vi "Overlay Arrow on Arc.vi"(5 "End Angle (degrees)":dbl format="%.2f", 6 "Scan Direction":u32(ring) items=["Counter-Clockwise", "Clockwise"], 7 "Start Angle (degrees)":dbl format="%.2f", 8 "error in (no error)":errorcluster, 9 "Color":u32(colorbox)=16711680, 10 "Bounding Rectangle":T2, 11 "Image":T1) -> (0 "error out":errorcluster, 3 "Image Out":T1)   [LabVIEW 2020]
uses:
  IMAQ Image.ctl
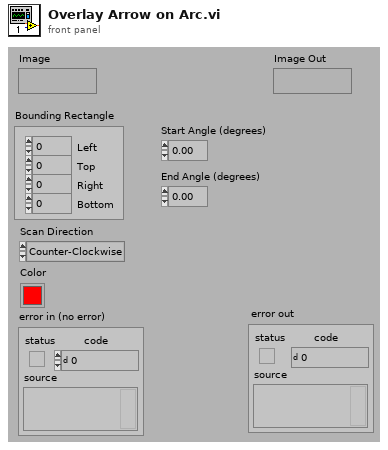
[diagram p1: front panel]
types:
  T1 = typedef "IMAQ Image.ctl" = refnum<image>
  T2 = cluster{"Left":i32, "Top":i32, "Right":i32, "Bottom":i32}
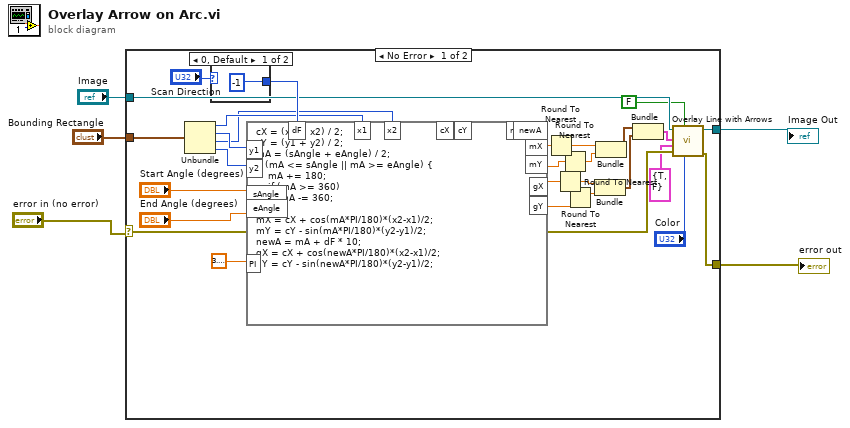
[diagram p0: block diagram]
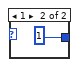
[diagram p2: hidden frame]
diagram:
  n1 = case shown="No Error" "error in (no error)" {
    selector: "error in (no error)" -> [w19 w36]
    tunnel: "Bounding Rectangle" -> [w32 _]
    tunnel: "Image" -> [w22 w37]
    tunnel: [w21 w37] -> w3
    tunnel: [w20 w36] -> w1
    frame No Error {
      n2 = Unbundle(w32) -> ("Left"=w30:i32, "Top"=w29:i32, "Right"=w27:i32, "Bottom"=w28:i32)
      n3 = case shown="0, Default" "Scan Direction" {
        tunnel: [-1 1] -> w31
        frame 0, Default {
        }
        frame 1 {
        }
      }
      n4 = formula code="cX = (x1 + x2) / 2;\ncY = (y1 + y2) / 2;\nmA = (sAngle + eAngle) / 2;\nif (mA <= sAngle || mA >= eAngle) {\n    mA += 180;\n    if (mA >= 360)\n        mA -= 360;\n}\nmX = cX + cos(mA*PI/180)*(x2-x1)/2;\nmY = cY - sin(mA*PI/180)*(y2-y1)/2;\nnewA = mA + dF * 10;\ngX = cX + cos(newA*PI/180)*(x2-x1)/2;\ngY = cY - sin(newA*PI/180)*(y2-y1)/2;"("x1"=w30, "x2"=w27, "y1"=w29, "y2"=w28, "sAngle"="Start Angle (degrees)", "eAngle"="End Angle (degrees)", "dF"=w31, "PI"=3.141592653589793) -> ("gX"=w18:dbl, "mX"=w17:dbl, "mY"=w16:dbl, "gY"=w15:dbl)  [unwired: 5 out]
      n5 = Round To Nearest(number=w17) -> (nearest integer value=w9:dbl)
      n6 = Round To Nearest(number=w18) -> (nearest integer value=w7:dbl)
      n7 = Round To Nearest(number=w16) -> (nearest integer value=w8:dbl)
      n8 = Round To Nearest(number=w15) -> (nearest integer value=w6:dbl)
      n9 = Bundle(w7, w6) -> (w13:cluster{dbl, dbl})  [unwired: 1 out]
      n10 = Bundle(w9, w8) -> (w14:cluster{dbl, dbl})  [unwired: 1 out]
      n11 = Bundle(w14, w13) -> (w12:cluster{cluster{dbl, dbl}, cluster{dbl, dbl}})  [unwired: 1 out]
      n12 = call "Overlay Line with Arrows.vi"("Color"="Color", "Draw line?"=FALSE, "error in (no error)"=w19, "Arrows"=cluster{"Start point":bool, "End point":bool} {"Start point"=TRUE, "End point"=FALSE}, "Line Coordinates"=w12, "Image In"=w22) -> ("error out"=w20:errorcluster, "Image Out"=w21:T1)  [unwired: 4 out]
    }
    frame Error {
    }
  }
  "error out" <- w1
  "Image Out" <- w3
